vi "Get File Extension.vi"(8 "error in (no error)":errorcluster, 11 "file":path) -> (0 "error out":errorcluster, 1 "filename without extension":string, 2 "lowercase file extension":string, 3 "dup file":path, 4 "unmodified file extension":string)   [LabVIEW 2026]
doc: "<p>Returns the file extension, without the period (.), of a file you specify.</p>"
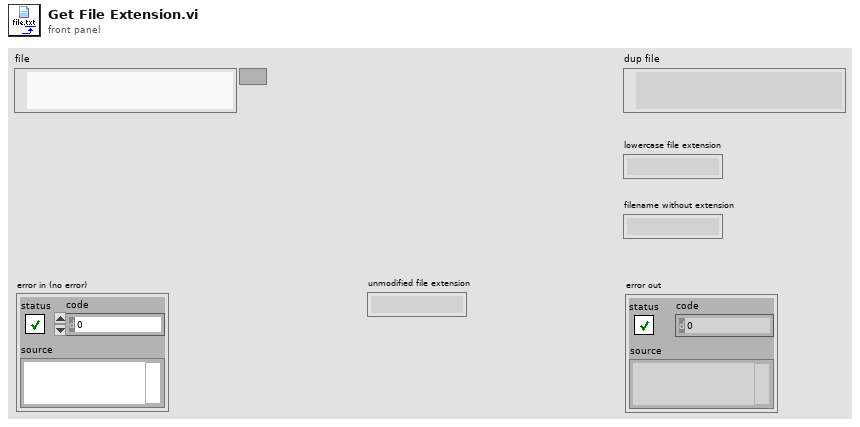
[diagram p1: front panel]
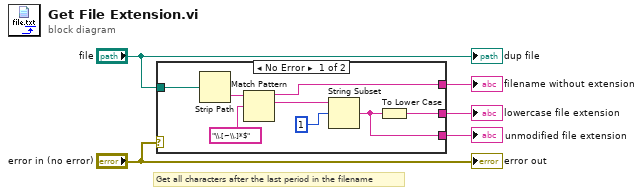
[diagram p0: block diagram]
diagram:
  # "Get all characters after the last period in the filename"
  n1 = case shown="No Error" "error in (no error)" {
    tunnel: "file" -> [w12 _]
    tunnel: [w10 _] -> w3
    tunnel: [w7 _] -> w2
    tunnel: [w6 _] -> w1
    frame No Error {
      n2 = Strip Path(path=w12) -> (name=w11:string)  [unwired: 1 out]
      n3 = Match Pattern(string=w11, regular expression="\\.[~\\.]*$") -> (before substring=w7:string, match substring=w13:string)  [unwired: 3 out]
      n4 = String Subset(string=w13, offset (0)=1) -> (substring=w6:string)  [unwired: 1 out]
      n5 = To Lower Case(string=w6) -> (all lower case string=w10:string)
    }
    frame Error {
    }
  }
  "lowercase file extension" <- w3
  "filename without extension" <- w2
  "unmodified file extension" <- w1
  "error out" <- "error in (no error)"
  "dup file" <- "file"
